vi "Make pulses.vi"(0 "phases":i32=3 caption="Phases", 1 "pulsedir":enum16{"Left", "Right", "Both"}(ring)=enum."Both" caption="Direction", 3 "pulsereps":i32=2 caption="Repetitions", 4 "Amplitudes":dbl[](array[numeric])=[5.0], 5 "Durations":dbl[](array[numeric])=[0.2], 6 "Output freq (Hz)":dbl=50.0 format="%#_13g", 7 "randomize":bool=TRUE, 8 "pre cycles":dbl=10.0 caption="Pre cycles", 9 "post cycles":dbl=10.0 caption="Post cycles", 10 "cyclesperpulse":dbl=10.0 caption="Cycles per pulse", 11 "sinfreq":dbl=1.5 caption="sinefreq", 13 "sinamp":dbl=20.0 caption="sineamp") -> (14 "pulse data":T2, 15 "sine signal":dbl[](array[numeric]), 17 "pulse signal":dbl[](array[numeric]), 18 "totaltime":dbl caption="Total time", 19 "stimphases":T1)   [LabVIEW 2013]
uses:
  Pulse data.ctl
  Phases.ctl
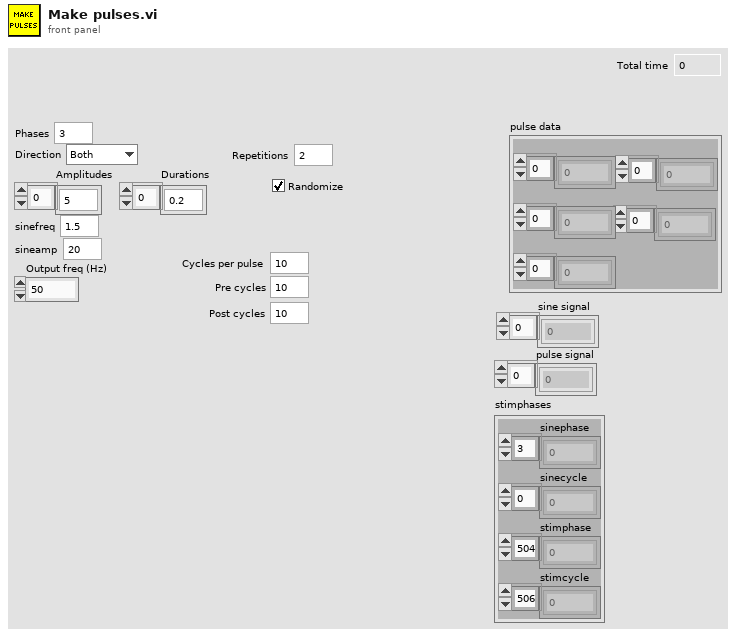
[diagram p1: front panel]
types:
  T1 = typedef "Phases.ctl" = cluster{"sinephase":dbl[], "sinecycle":dbl[], "stimphase":dbl[], "stimcycle":dbl[]}
  T2 = typedef "Pulse data.ctl" = cluster{"time":dbl[], "phase":dbl[], "dir/phase2":dbl[], "amplitude":dbl[], "duration":dbl[]}
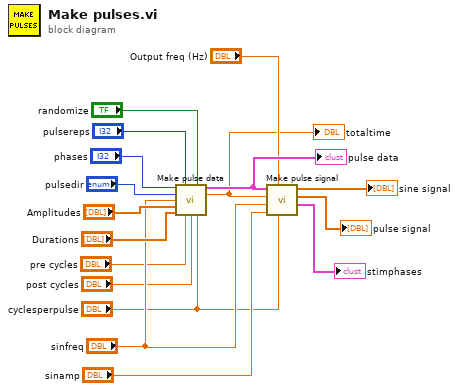
[diagram p0: block diagram]
diagram:
  n1 = call "Make pulse data.vi"("phases"="phases", "pulsereps"="pulsereps", "randomize"="randomize", "pulsedir"="pulsedir", "sinfreq"="sinfreq", "Amplitudes"="Amplitudes", "Durations"="Durations", "pre cycles"="pre cycles", "post cycles"="post cycles", "cyclesperpulse"="cyclesperpulse") -> ("pulse data"=w13:T2, "totaltime"=w7:dbl)  [unwired: 4 in]
  "pulse data" <- w13
  "totaltime" <- w7
  n2 = call "Make pulse signal.vi"("cyclesperpulse"="cyclesperpulse", "Output freq (Hz)"="Output freq (Hz)", "sinamp"="sinamp", "sinfreq"="sinfreq", "total time"=w7, "pulse data"=w13) -> ("phases"=→"stimphases":T1, "pulse signal"=→"pulse signal":dbl[], "sine signal"=→"sine signal":dbl[])  [unwired: 3 in]
